vi "Util_RT_ElapsedTimer.vi"(8 "Pause":bool, 9 "Reset":bool, 10 "Auto Reset":bool=TRUE, 11 "Target Time (s)":dbl=1.0) -> (2 "Target\nReached":bool, 3 "Timer (s)":dbl)   [LabVIEW 2019]
doc: "Generic timer with pause, reset, and auto reset capability. Target Time has double precision and units of seconds."
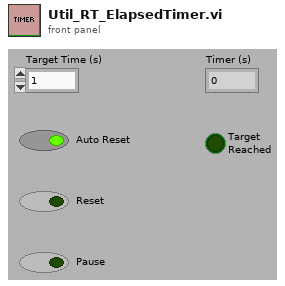
[diagram p1: front panel]
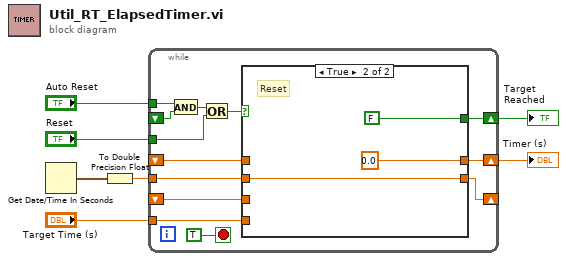
[diagram p0: block diagram]
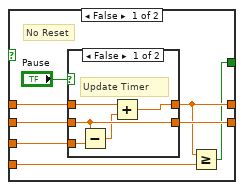
[diagram p2: hidden frame]
diagram:
  n1 = Get Date/Time In Seconds() -> (seconds since 1Jan1904=w7:timestamp)
  n2 = To Double Precision Float(number=w7) -> (double precision float=w3:dbl)
  n3 = while {
    tunnel: "Reset" -> [w11]
    shift-right: [w19] -> w5
    shift-left: _ -> [w17]
    tunnel: w3 -> [w15]
    shift-right: [w16] -> _
    shift-left: _ -> [w14]
    tunnel: "Target Time (s)" -> [w13]
    shift-right: [w18] -> w4
    shift-left: _ -> [w8]
    tunnel: "Auto Reset" -> [w9]
    stop <- TRUE stop-if-true
    n4 = And(x=w9, y=w8) -> (x .and. y?=w12:bool)
    n5 = Or(x=w12, y=w11) -> (x .or. y?=w10:bool)
    n6 = case shown="True" w10 {
      tunnel: [w24 0.0] -> w19
      tunnel: [w22 FALSE] -> w18
      tunnel: w17 -> [w28 _]
      tunnel: [w27 w36] -> w16
      tunnel: w15 -> [w26 w36]
      tunnel: w14 -> [w25 _]
      tunnel: w13 -> [w23 _]
      frame False {
        # "No Reset"
        n7 = case shown="False" "Pause" {
          tunnel: [w29 w35] -> w24
          tunnel: w28 -> [w31 w35]
          tunnel: [w33 w34] -> w27
          tunnel: w26 -> [w33 w34]
          tunnel: w25 -> [w32 _]
          frame False {
            # "Update Timer"
            n8 = Subtract(x=w33, y=w32) -> (x-y=w30:dbl)
            n9 = Add(x=w31, y=w30) -> (x+y=w29:dbl)
          }
          frame True {
            # "No Update"
          }
        }
        n10 = Greater Or Equal?(x=w24, y=w23) -> (x >= y?=w22:bool)
      }
      frame True {
        # "Reset"
      }
    }
  }
  "Target\nReached" <- w4
  "Timer (s)" <- w5
